vi "Abort Connection Loop.vi"(8 "error in (no error)":errorcluster, 11 "TCP Client in":refnum<class "TCP Client.lvclass">) -> (0 "error out":errorcluster, 3 "TCP Client out":refnum<class "TCP Client.lvclass">)   [LabVIEW 2020, in "Stream-TCP.lvlib" / "TCP Client.lvclass"]
uses:
  TCP Client.lvclass
  Connection State.ctl
  TCP Client.lvclass/TCP Client.ctl
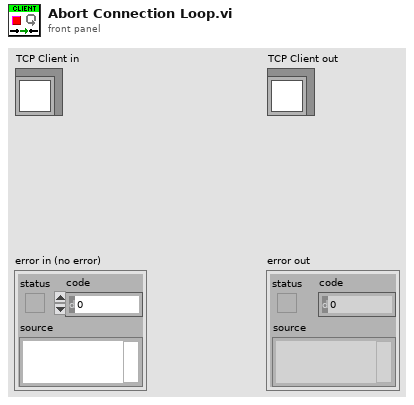
[diagram p1: front panel]
types:
  T1 = typedef "Stream-TCP.lvlib/TCP Client.lvclass/Connection State.ctl" = enum16{"Closed", "Idle", "Connecting", "Connected", "Shutdown"}
  T2 = typedef "Stream-TCP.lvlib/TCP Client.lvclass/Ref Data.ctl" = cluster{"TCP Connection":refnum<k5>, "TCP Stream":refnum<class "TCP Stream.lvclass">, "State":T1, "Connection Loop":refnum<vi>, "TCP Mode":T3, "Timeout ms":i32, "Server Connection":bool}
  T3 = typedef "Stream-TCP.lvlib/TCP Mode.ctl" = enum16{"buffered", "raw"}
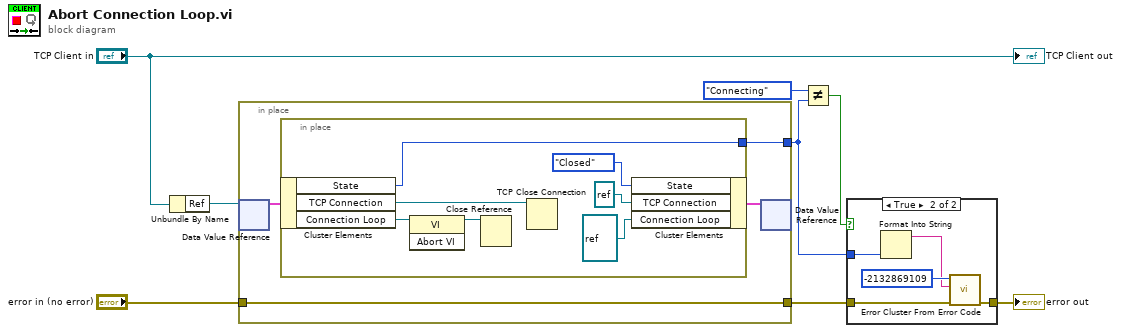
[diagram p0: block diagram]
diagram:
  n1 = Unbundle By Name("TCP Client in") -> ("Ref"=w8:refnum<data-value>)
  n2 = in-place {
    in-place-border: [w10] -> w5
    in-place-border: "error in (no error)" -> [w9]
    in-place-border: [w9] -> w2
    n3 = in-place-dvr #1(w8) -> (w12:T2)  [unwired: 1 out]
    n4 = in-place {
      in-place-border: [w14] -> w10
      n5 = in-place-cluster #2(w12) -> ("State"=w14:T1, "TCP Connection"=w16:refnum<k5>, "Connection Loop"=w17:refnum<vi>)
      n6 = invoke class="VI" method="Abort VI"(reference=w17) -> (reference out=w13:refnum<vi>)  [unwired: 2 in, 2 out]
      n7 = Close Reference(reference=w13) -> ()  [unwired: 1 in, 1 out]
      n8 = TCP Close Connection(connection ID=w16) -> ()  [unwired: 2 in, 2 out]
      n9 = in-place-cluster #2("State"=Connection_State."Closed", "TCP Connection"=refnum<k5> refnum, "Connection Loop"=refnum<vi> refnum) -> (w11:T2)
    }
    n10 = in-place-dvr #1(w11) -> ()  [unwired: 2 out]
  }
  n11 = Not Equal?(x=Connection_State."Connecting" ("State"), y=w5) -> (x != y?=w4:bool)
  n12 = case shown="True" w4 {
    tunnel: w2 -> [w20 w24]
    tunnel: w5 -> [_ w23]
    tunnel: [w20 w21] -> w1
    frame False {
    }
    frame True {
      n13 = Format Into String(w23) -> (resulting string=w22:string)  [unwired: 3 in, 1 out]
      n14 = call <vilib>:"Error Cluster From Error Code.vi"("error in (no error)"=w24, "error message (\"\")"=w22, "error code (0)"=-2132869109) -> ("error out"=w21:errorcluster)  [unwired: 6 in]
    }
  }
  "error out" <- w1
  "TCP Client out" <- "TCP Client in"
